vi "GetStabilizedPressureData.vi"(6 "Graph in":cluster{dbl[], dbl[]}, 7 "WaitTime":i32, 8 "error in":errorcluster, 9 "SampleCount":i32, 10 "Variance/Mean Trigger":dbl, 11 "MinimalWaitTimems":u32) -> (0 "error out":errorcluster, 2 "Values":cluster{dbl[], dbl[]}, 3 "StabilityAchieved":bool)   [LabVIEW 2013]
uses:
  GlobalVariables/AllowContinuousPressureAcquisition.vi
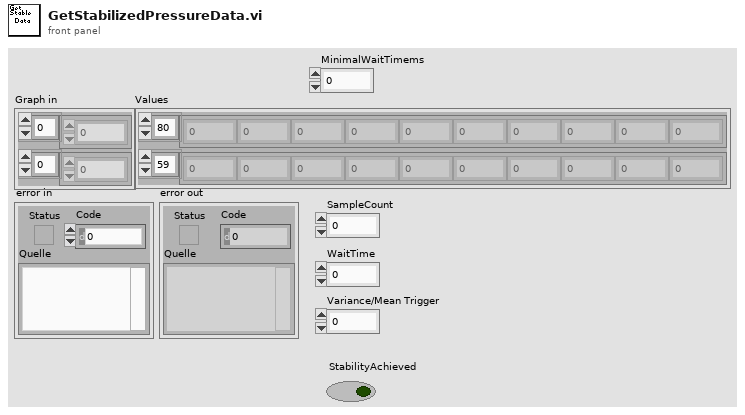
[diagram p1: front panel]
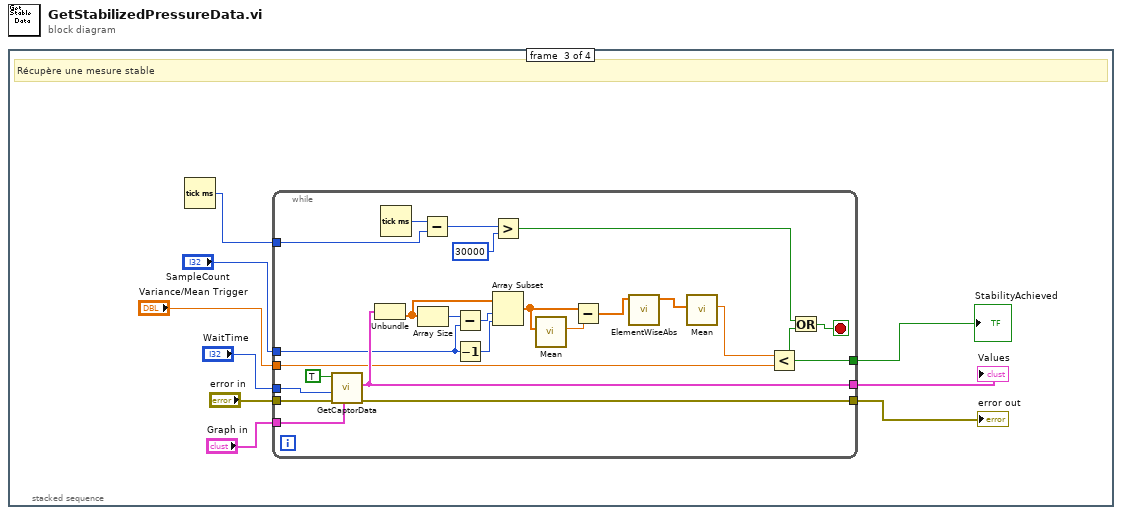
[diagram p0: block diagram]
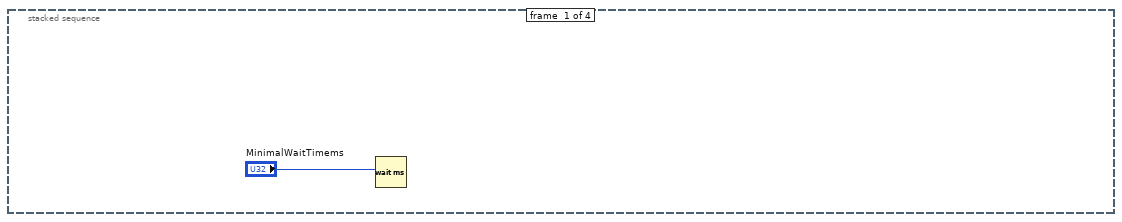
[diagram p2: hidden frame]
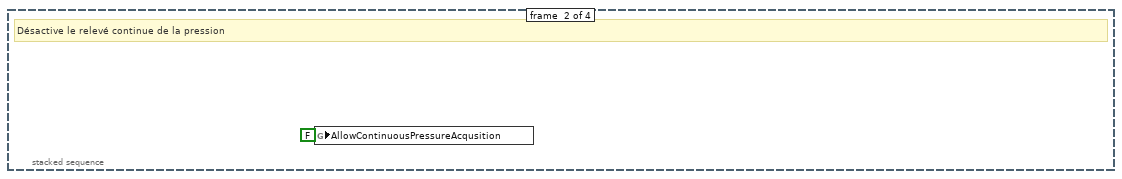
[diagram p3: hidden frame]
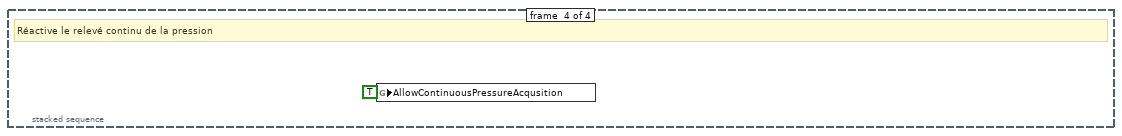
[diagram p4: hidden frame]
diagram:
  n1 = stacked-sequence {
    frame #0 {
      n2 = Wait (ms)(milliseconds to wait="MinimalWaitTimems") -> ()  [unwired: 1 out]
    }
    frame #1 {
      # "Désactive le relevé continue de la pression"
      n3 = global write "AllowContinuousPressureAcquisition.vi" "AllowContinuousPressureAcqusition"(FALSE) -> ()
    }
    frame #2 {
      # "Récupère une mesure stable"
      n4 = Tick Count (ms)() -> (millisecond timer value=w4:u32)
      n5 = while {
        tunnel: "error in" -> [w29]
        tunnel: [w28] -> w8
        tunnel: "Graph in" -> [w34]
        tunnel: [w30] -> w10
        tunnel: "SampleCount" -> [w24]
        tunnel: "Variance/Mean Trigger" -> [w26]
        tunnel: "WaitTime" -> [w27]
        tunnel: w4 -> [w17]
        tunnel: [w12] -> w3
        stop <- w14 stop-if-true
        n6 = call "GetCaptorData.vi"("Graph in"=w34, "error in"=w29, "Length"=w27, "ON"=TRUE) -> ("error out"=w28:errorcluster, "Values"=w30:cluster{dbl[], dbl[]})  [unwired: 6 in]
        n7 = Unbundle(w30) -> (w33:dbl[])  [unwired: 1 out]
        n8 = Tick Count (ms)() -> (millisecond timer value=w18:u32)
        n9 = Array Size(array=w33) -> (size(s)=w32:i32)
        n10 = Subtract(x=w18, y=w17) -> (x-y=w16:u32)
        n11 = Subtract(x=w32, y=w24) -> (x-y=w31:i32)
        n12 = Decrement(x=w24) -> (x-1=w22:i32)
        n13 = Greater?(x=w16, y=u32 30000 ("x")) -> (0:w13:bool)
        n14 = Array Subset(array=w33, index=w31, length=w22) -> (w25:dbl[])
        n15 = call "Mean.vi"("Array"=w25) -> ("Mean"=w23:dbl)  [unwired: 10 in]
        n16 = Subtract(x=w25, y=w23) -> (x-y=w21:dbl[])
        n17 = call "ElementWiseAbs.vi"("Array [in]"=w21) -> ("Array[out]"=w20:dbl[])  [unwired: 10 in]
        n18 = call "Mean.vi"("Array"=w20) -> ("Mean"=w19:dbl)  [unwired: 10 in]
        n19 = Less?(x=w19, y=w26) -> (x < y?=w12:bool)
        n20 = Or(x=w13, y=w12) -> (x .or. y?=w14:bool)
      }
      "Values" <- w10
      "error out" <- w8
      "StabilityAchieved" <- w3
    }
    frame #3 {
      # "Réactive le relevé continu de la pression"
      n21 = global write "AllowContinuousPressureAcquisition.vi" "AllowContinuousPressureAcqusition"(TRUE) -> ()
    }
  }
